vi "nD B-Spline Fit.vi"(0 "Data":dbl[][](array[numeric]), 1 "# of control points":i32=10, 7 "Weight":dbl[](array[numeric]), 12 "degree":i32=3, 13 "parameter selection":u16(ring)=2 items=["equally spaced", "chord length", "centripetal"]) -> (4 "Best BSpline Fit":dbl[][](array[numeric]), 14 "residue":dbl, 15 "error":i32)   [LabVIEW 2017, in "NI_AALPro.lvlib"]
uses:
  NI_AALPro.lvlib
panel:
  # "nD B-Spline Fit"
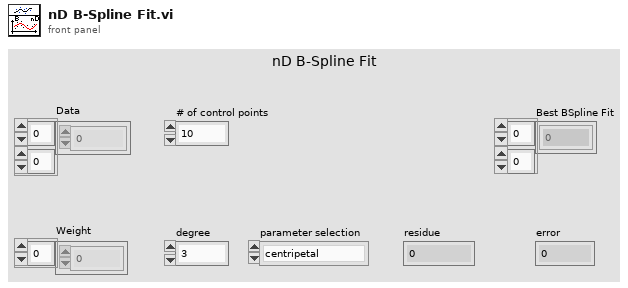
[diagram p1: front panel]
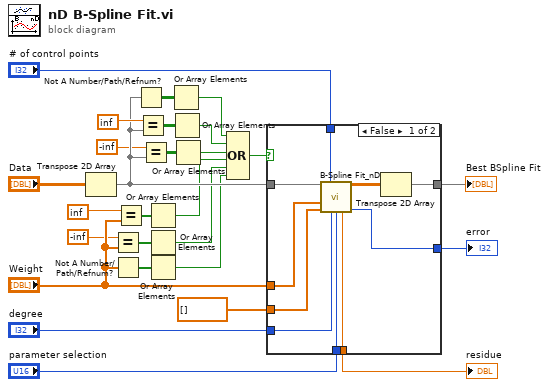
[diagram p0: block diagram]
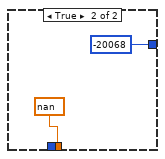
[diagram p2: hidden frame]
diagram:
  n1 = Transpose 2D Array(2D array="Data") -> (transposed array=w12:dbl[][])
  n2 = Equal?(x=-inf, y="Weight") -> (x = y?=w14:bool[])
  n3 = Not A Number/Path/Refnum?(number/path/refnum="Weight") -> (NaN/Path/Refnum?=w19:bool[])
  n4 = Equal?(x=inf, y="Weight") -> (x = y?=w13:bool[])
  n5 = Not A Number/Path/Refnum?(number/path/refnum=w12) -> (NaN/Path/Refnum?=w20:bool[][])
  n6 = Equal?(x=inf, y=w12) -> (x = y?=w17:bool[][])
  n7 = Equal?(x=-inf, y=w12) -> (x = y?=w10:bool[][])
  n8 = Or Array Elements(Boolean array=w13) -> (logical OR=w5:bool)
  n9 = Or Array Elements(Boolean array=w14) -> (logical OR=w4:bool)
  n10 = Or Array Elements(Boolean array=w19) -> (logical OR=w3:bool)
  n11 = Or Array Elements(Boolean array=w20) -> (logical OR=w8:bool)
  n12 = Or Array Elements(Boolean array=w17) -> (logical OR=w7:bool)
  n13 = Or Array Elements(Boolean array=w10) -> (logical OR=w6:bool)
  n14 = Compound Arithmetic op=OR(w8, w7, w6, w5, w4, w3) -> (w2:bool)
  n15 = case shown="False" w2 {
    tunnel: "# of control points" -> [w37 _]
    tunnel: "degree" -> [w36 _]
    tunnel: [w35 nan ("residue")] -> w25
    tunnel: "parameter selection" -> [w34 _]
    tunnel: [w33 -20068 ("error")] -> w23
    tunnel: "Weight" -> [w32 _]
    tunnel: w12 -> [w31 _]
    tunnel: dbl[] [] ("parameter") -> [w30 _]
    tunnel: [w28 _] -> w1
    frame False {
      n16 = call "B-Spline Fit_nD.vi"("Y"=w31, "# of control points"=w37, "Weight"=w32, "Parameter"=w30, "degree"=w36, "parameter selection"=w34) -> ("BSpline fit Y"=w29:dbl[][], "residue"=w35:dbl, "error"=w33:i32)  [unwired: 7 out]
      n17 = Transpose 2D Array(2D array=w29) -> (transposed array=w28:dbl[][])
    }
    frame True {
    }
  }
  "error" <- w23
  "residue" <- w25
  "Best BSpline Fit" <- w1
